vi "FindPicturesFolderFromRawData.vi"(11 "RawDataFile":path) -> (1 "RawDataName":string, 2 "PicturesPath":path)   [LabVIEW 2015]
doc: "Finds the location of the Pictures folder for a given RawDataFile"
panel:
  # "Finds the location of the Pictures folder for a given RawDataFile"
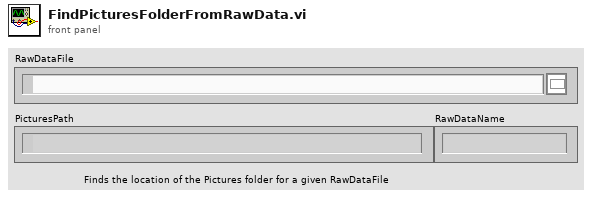
[diagram p1: front panel]
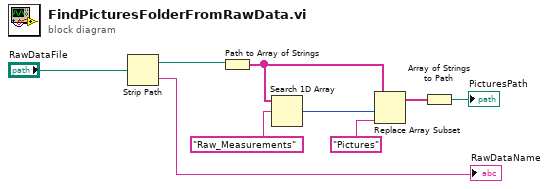
[diagram p0: block diagram]
diagram:
  n1 = Strip Path(path="RawDataFile") -> (stripped path=w4:path, name=→"RawDataName":string)
  n2 = Path to Array of Strings(0:w4) -> (2:w7:string[])  [unwired: 1 out]
  n3 = Search 1D Array(1D array=w7, element="Raw_Measurements") -> (index of element=w6:i32)  [unwired: 1 in]
  n4 = Replace Array Subset(array=w7, new element="Pictures", index=w6) -> (w3:string[])
  n5 = Array of Strings to Path(0:w3) -> (2:→"PicturesPath":path)  [unwired: 1 in]
